vi "GlobalAcquireFocusFlag.vi"() -> ()   [LabVIEW 2010]
panel:
  in  "AcquireFocusFlag":u32
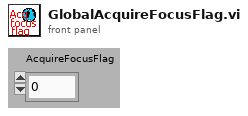
[diagram p1: front panel]
diagram:
